vi "ConfigureGalvos.vi"() -> ()   [LabVIEW 2017]
uses:
  classes/HardwareObjects/Galvonometer/Galvonometer.lvclass
  classes/HardwareObjects/DAQ/DAQ.lvclass
  classes/HardwareObjects/Galvonometer/Galvonometer.lvclass/Galvonometer.ctl
  classes/HardwareObjects/DAQ/DAQ.lvclass/DAQ.ctl
  classes/HardwareObjects/Galvonometer/Write Analog Output Channel.vi
  classes/HardwareObjects/Galvonometer/Write Make Model.vi
  classes/HardwareObjects/Galvonometer/Write Max Scan Angle (degrees).vi
  classes/HardwareObjects/Galvonometer/Write Output Scale Factor (V_degrees).vi
  classes/HardwareObjects/Galvonometer/Write Scan Direction.vi
  classes/HardwareObjects/Galvonometer/Read Analog Output Channel.vi
  classes/HardwareObjects/DAQ/Write Galvo Analog Output Channel(s).vi
panel:
  in  "Cancel":bool
  out "Updated DAQ":refnum<class "DAQ.lvclass">
  in  "DAQ.lvclass":refnum<class "DAQ.lvclass">
  out "Updated Galvo Array":refnum<class "Galvonometer.lvclass">[](array[class])
  in  "Galvo\nProperties":T1(array[cluster])=[{"Analog Output Channel"="Dev1/ao0", "Make Model"="TL GVS102", "Max Scan Angle (degrees)"=12.5, "Output Scale Factor (V/degrees)"=0.5, "Scan Direction"="X"}, {"Analog Output Channel"="Dev1/ao1", "Make Model"="TL GVS102", "Max Scan Angle (degrees)"=12.5, "Output Scale Factor (V/degrees)"=0.5, "Scan Direction"="Y"}]
  in  "Default\nGalvonometer":refnum<class "Galvonometer.lvclass">
  in  "OK":bool
  in  "Number of\nGalvos":u8=2 min=1 max=2 step=1
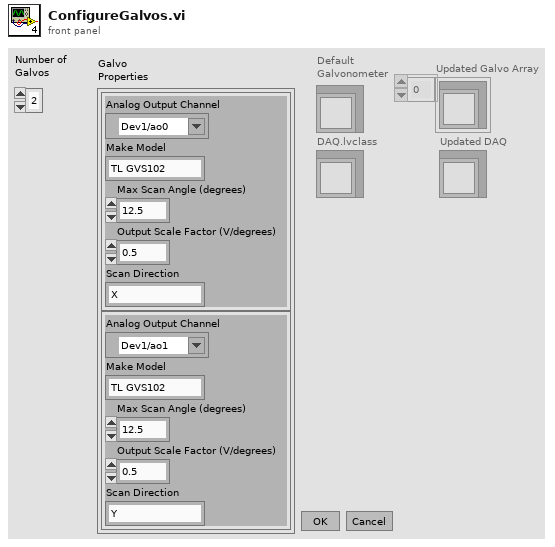
[diagram p1: front panel]
types:
  T1 = cluster{"Analog Output Channel":tag, "Make Model":string, "Max Scan Angle (degrees)":dbl, "Output Scale Factor (V/degrees)":dbl, "Scan Direction":string}[]
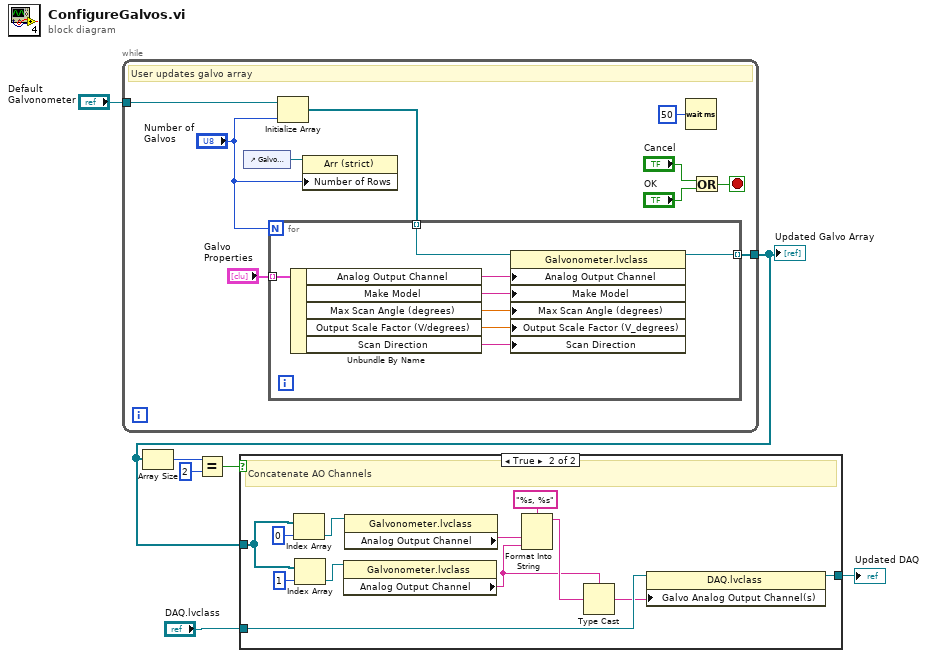
[diagram p0: block diagram]
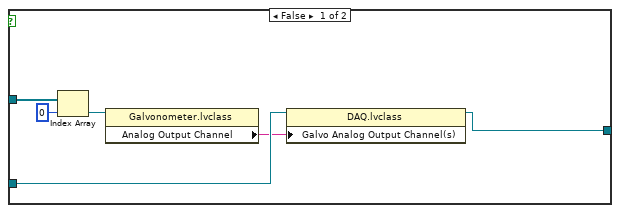
[diagram p2: hidden frame]
diagram:
  n1 = while {
    tunnel: "Default\nGalvonometer" -> [w12]
    tunnel: [w11] -> w3
    stop <- w8 stop-if-true
    # "User updates galvo array"
    n2 = control-ref of="Galvo\nProperties"() -> (w16:refnum<vi>)
    n3 = Initialize Array(w12, "Number of\nGalvos") -> (w13:refnum<class "Galvonometer.lvclass">[])
    n4 = for {
      N: "Number of\nGalvos" -> [_]
      tunnel: "Galvo\nProperties" -> [w24] mode=indexing
      tunnel: w13 -> [w25] mode=indexing
      tunnel: [w18] -> w11 mode=indexing
      n5 = Unbundle By Name(w24) -> ("Analog Output Channel"=w23:tag, "Make Model"=w22:string, "Max Scan Angle (degrees)"=w21:dbl, "Output Scale Factor (V/degrees)"=w20:dbl, "Scan Direction"=w19:string)
      n6 = property class="Galvonometer.lvclass"(reference=w25, "Analog Output Channel"=w23, "Make Model"=w22, "Max Scan Angle (degrees)"=w21, "Output Scale Factor (V_degrees)"=w20, "Scan Direction"=w19) -> (reference out=w18:refnum<class "Galvonometer.lvclass">)  [unwired: 1 in, 1 out]
    }
    n7 = property class="Arr (strict)"(reference=w16, "Number of Rows"="Number of\nGalvos") -> ()  [unwired: 1 in, 2 out]
    n8 = Wait (ms)(milliseconds to wait=u32 50) -> ()  [unwired: 1 out]
    n9 = Or(x="Cancel", y="OK") -> (x .or. y?=w8:bool)
  }
  "Updated Galvo Array" <- w3
  n10 = Array Size(array=w3) -> (size(s)=w6:i32)
  n11 = Equal?(x=w6, y=2) -> (x = y?=w4:bool)
  n12 = case shown="True" w4 {
    tunnel: w3 -> [w31 w39]
    tunnel: "DAQ.lvclass" -> [w28 w34]
    tunnel: [w26 w32] -> w1
    frame False {
      n13 = Index Array(array=w31, index=0) -> (element=w29:refnum<class "Galvonometer.lvclass">)
      n14 = property class="Galvonometer.lvclass"(reference=w29) -> ("Analog Output Channel"=w27:tag)  [unwired: 1 in, 2 out]
      n15 = property class="DAQ.lvclass"(reference=w28, "Galvo Analog Output Channel(s)"=w27) -> (reference out=w26:refnum<class "DAQ.lvclass">)  [unwired: 1 in, 1 out]
    }
    frame True {
      # "Concatenate AO Channels"
      n16 = Index Array(array=w39, index=0) -> (element=w38:refnum<class "Galvonometer.lvclass">)
      n17 = Index Array(array=w39, index=1) -> (element=w37:refnum<class "Galvonometer.lvclass">)
      n18 = property class="Galvonometer.lvclass"(reference=w37) -> ("Analog Output Channel"=w35:tag)  [unwired: 1 in, 2 out]
      n19 = property class="Galvonometer.lvclass"(reference=w38) -> ("Analog Output Channel"=w42:tag)  [unwired: 1 in, 2 out]
      n20 = Format Into String(format string="%s, %s", w42, w35) -> (resulting string=w36:string)  [unwired: 2 in, 1 out]
      n21 = Type Cast(type=w35, x=w36) -> (*(type *) &x=w33:tag)
      n22 = property class="DAQ.lvclass"(reference=w34, "Galvo Analog Output Channel(s)"=w33) -> (reference out=w32:refnum<class "DAQ.lvclass">)  [unwired: 1 in, 1 out]
    }
  }
  "Updated DAQ" <- w1
